vi "Do.vi"(8 "error in (no error)":errorcluster, 10 "Actor in":refnum<class "Actor.lvclass">, 11 "Message":refnum<class "Iteration Msg.lvclass">) -> (0 "error out":errorcluster, 2 "Actor out":refnum<class "Actor.lvclass">)   [LabVIEW 2023, in "Example Iterator NR Actor.lvlib" / "Iteration Msg.lvclass"]
doc: "(<B>Filename</B>: Actor Framework.lvlib:Reply Msg.lvclass:Do Core.vi)\n\nDefines what an actor does when it receives <B>Reply Message</B>. This method also defines the <B>Reply</B> that is returned to the actor that sent <B>Reply Message</B>.\n\nBy default, this method does nothing, and <B>Reply</B> is the ancestor Message class. A child class must override this method to define behavior and specify a child of the Message class to return in the <B>Reply</B> output."
uses:
  Iteration Msg.lvclass
  <vilib>/ActorFramework/Actor/Actor.lvclass
  Example Actor/Example Actor.lvclass
  C:/Program Files/National Instruments/LabVIEW 2023/vi.lib/ActorFramework/Actor/Actor.lvclass
  Iteration Msg.lvclass/Iteration Msg.ctl
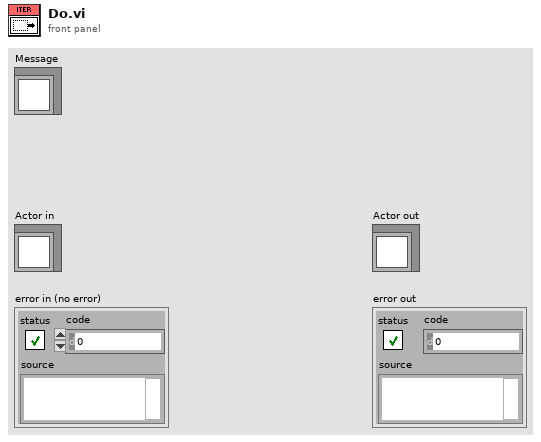
[diagram p1: front panel]
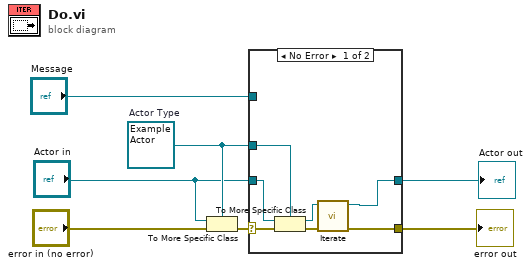
[diagram p0: block diagram]
diagram:
  w6 = refnum<class "Example Actor.lvclass"> refnum  # Actor Type
  n1 = To More Specific Class(target class=w6, reference="Actor in", error in="error in (no error)") -> (error out=w7:errorcluster)  [unwired: 1 out]
  n2 = case shown="No Error" w7 {
    selector: w7 -> [w14 w16]
    tunnel: [w9 w16] -> w2
    tunnel: [w8 w15] -> w3
    tunnel: "Actor in" -> [w13 w15]
    tunnel: w6 -> [w12 _]
    tunnel: "Message" -> [_ _]
    frame No Error {
      n3 = To More Specific Class ("Actor Cast")(target class=w12, reference=w13, error in=w14) -> (specific class reference=w11:refnum<class "Example Actor.lvclass">, error out=w10:errorcluster)
      n4 = call "Iterate.vi"("error in (no error)"=w10, "Example Actor in"=w11) -> ("error out"=w9:errorcluster, "Example Actor out"=w8:refnum<class "Example Actor.lvclass">)  [unwired: 8 in]
    }
    frame Error {
    }
  }
  "error out" <- w2
  "Actor out" <- w3
